vi "Rear Rocket to Score.vi"() -> (4 "path":cluster{"X":dbl, "Y":dbl}[](array[cluster])=[{"X"=300.0, "Y"=62.0}, {"X"=299.67796585022535, "Y"=61.06513991194655}, {"X"=299.35531113454925, "Y"=60.131107487190775}, {"X"=299.0313812985895, "Y"=59.19877965387899}, {"X"=298.7054549995574, "Y"=58.26912580374255}, {"X"=298.376704877581, "Y"=57.343252442862465}, {"X"=298.04415663192685, "Y"=56.42246009840396}, {"X"=297.70664011718065, "Y"=55.50831518041174}, {"X"=297.3627267868247, "Y"=54.602736376469785}, {"X"=297.010650930695, "Y"=53.708096849775444}, {"X"=296.64821357013733, "Y"=52.82734746493497}, {"X"=296.2726661277642, "Y"=51.96416944345233}, {"X"=295.88056891520927, "Y"=51.123167538744006}, {"X"=295.4676069213577, "Y"=50.31010763033021}, {"X"=295.0283908833696, "Y"=49.532242809593704}, {"X"=294.5560954613462, "Y"=48.7986359651749}, {"X"=294.0284648626625, "Y"=48.0784796591909}, {"X"=293.4567720099731, "Y"=47.36905297576079}, {"X"=292.85006167096424, "Y"=46.66825385588848}, {"X"=292.21553026302087, "Y"=45.9744402337975}, {"X"=291.5588656657838, "Y"=45.28630800332636}, {"X"=290.8846000891376, "Y"=44.60285095835355}, {"X"=290.196364261339, "Y"=43.92332453368775}, {"X"=289.49705315511903, "Y"=43.24719469139753}, {"X"=288.7889647280253, "Y"=42.574098303654296}, {"X"=288.0739306067003, "Y"=41.90382692056283}, {"X"=287.35342424819305, "Y"=41.23632388947038}, {"X"=286.6286381471462, "Y"=40.57168374443791}, {"X"=285.90053857777383, "Y"=39.91015312672445}, {"X"=285.1699127607743, "Y"=39.2521400561977}, {"X"=284.43740364738807, "Y"=38.59822952777461}, {"X"=283.70358294426364, "Y"=37.949238228876666}, {"X"=282.9688855497176, "Y"=37.30619626764946}, {"X"=282.2338323047616, "Y"=36.670539509494894}, {"X"=281.4987765734628, "Y"=36.04397819113178}, {"X"=280.7641553421933, "Y"=35.42878692701308}, {"X"=280.03044421363336, "Y"=34.827824744652226}, {"X"=279.2981146207875, "Y"=34.24466579102106}, {"X"=278.56770897603565, "Y"=33.68383375390436}, {"X"=277.8399028708086, "Y"=33.151044376258625}, {"X"=277.0852340691614, "Y"=32.62621063659758}, {"X"=276.3096142473145, "Y"=32.10793481435018}, {"X"=275.51783999700325, "Y"=31.59516350001117}, {"X"=274.71386264087107, "Y"=31.087138412194943}, {"X"=273.9010019494029, "Y"=30.583354256294154}, {"X"=273.0821128441466, "Y"=30.08352650030417}, {"X"=272.2597284445897, "Y"=29.58757798169254}, {"X"=271.43618730520296, "Y"=29.095626058533444}, {"X"=270.6137768577266, "Y"=28.60801853264354}, {"X"=269.7948293153701, "Y"=28.125304207113395}, {"X"=268.9818874214875, "Y"=27.648321209906022}, {"X"=268.17779535712015, "Y"=27.17819420680734}, {"X"=267.3858611746366, "Y"=26.716401759600387}, {"X"=266.61003761727807, "Y"=26.26486982962313}, {"X"=265.85512070414063, "Y"=25.82606549423999}, {"X"=265.1270026053729, "Y"=25.40312036911472}, {"X"=264.4329896907217, "Y"=25.0}], 6 "Reverse Path?":bool)   [LabVIEW 2018]
uses:
  AutonBuilder/Typedef/Data Point.ctl
panel:
  in  "Data Points":T1[](array[typedef])=[{"X"=300.0, "Y"=62.0, "Theta"=0.0, "Speed %"=0.0, "Disabled?"=FALSE}, {"X"=295.60824742268045, "Y"=48.54355400696864, "Theta"=0.0, "Speed %"=0.0, "Disabled?"=FALSE}, {"X"=278.35051546391753, "Y"=33.0, "Theta"=0.0, "Speed %"=0.0, "Disabled?"=FALSE}, {"X"=264.4329896907217, "Y"=25.0, "Theta"=0.0, "Speed %"=0.0, "Disabled?"=FALSE}]
  out "Graph":cluster{dbl[], dbl[]}[](graph)=[{[280.5, 314.0, 314.0, 280.5, 280.5], [76.25, 76.25, 47.75, 47.75, 76.25]}, {[300.0, 295.60824742268045, 278.35051546391753, 264.4329896907217], [62.0, 48.54355400696864, 33.0, 25.0]}, {[300.0, 299.67796585022535, 299.35531113454925, 299.0313812985895, 298.7054549995574, 298.376704877581, 298.04415663192685, 297.70664011718065, 297.3627267868247, 297.010650930695, 296.64821357013733, 296.2726661277642, 295.88056891520927, 295.4676069213577, 295.0283908833696, 294.5560954613462, 294.0284648626625, 293.4567720099731, 292.85006167096424, 292.21553026302087, 291.5588656657838, 290.8846000891376, 290.196364261339, 289.49705315511903, 288.7889647280253, 288.0739306067003, 287.35342424819305, 286.6286381471462, 285.90053857777383, 285.1699127607743, 284.43740364738807, 283.70358294426364, 282.9688855497176, 282.2338323047616, 281.4987765734628, 280.7641553421933, 280.03044421363336, 279.2981146207875, 278.56770897603565, 277.8399028708086, 277.0852340691614, 276.3096142473145, 275.51783999700325, 274.71386264087107, 273.9010019494029, 273.0821128441466, 272.2597284445897, 271.43618730520296, 270.6137768577266, 269.7948293153701, 268.9818874214875, 268.17779535712015, 267.3858611746366, 266.61003761727807, 265.85512070414063, 265.1270026053729, 264.4329896907217], [62.0, 61.06513991194655, 60.131107487190775, 59.19877965387899, 58.26912580374255, 57.343252442862465, 56.42246009840396, 55.50831518041174, 54.602736376469785, 53.708096849775444, 52.82734746493497, 51.96416944345233, 51.123167538744006, 50.31010763033021, 49.532242809593704, 48.7986359651749, 48.0784796591909, 47.36905297576079, 46.66825385588848, 45.9744402337975, 45.28630800332636, 44.60285095835355, 43.92332453368775, 43.24719469139753, 42.574098303654296, 41.90382692056283, 41.23632388947038, 40.57168374443791, 39.91015312672445, 39.2521400561977, 38.59822952777461, 37.949238228876666, 37.30619626764946, 36.670539509494894, 36.04397819113178, 35.42878692701308, 34.827824744652226, 34.24466579102106, 33.68383375390436, 33.151044376258625, 32.62621063659758, 32.10793481435018, 31.59516350001117, 31.087138412194943, 30.583354256294154, 30.08352650030417, 29.58757798169254, 29.095626058533444, 28.60801853264354, 28.125304207113395, 27.648321209906022, 27.17819420680734, 26.716401759600387, 26.26486982962313, 25.82606549423999, 25.40312036911472, 25.0]}, {[302.86466642002404, 286.2049296430795, 285.8863016143085, 285.5706984813838, 285.25794442422927, 284.9480898615065, 284.64144909579124, 284.33869923581494, 284.04105177421627, 283.75052314685786, 283.470370216165, 283.20581673896623, 282.9652805494417, 282.76247671309693, 282.6198192416317, 282.57443861469056, 282.5335104549795, 282.3611354437252, 282.0765565739421, 281.70003519026403, 281.2496358321106, 280.7403468790285, 280.18445756578194, 279.59201059374533, 278.9711237054457, 278.3283352571779, 277.6689893589384, 276.99757110000064, 276.31795020342184, 275.6335640622988, 274.94761135851314, 274.2631927751518, 273.5836926739073, 272.9127122773153, 272.254686832191, 271.6151631816832, 271.0009291706447, 270.42133708095275, 269.8892351862872, 269.4225804954357, 268.9491661733871, 268.39249314054535, 267.771752324279, 267.101785832785, 266.39415115658835, 265.65798842977506, 264.9007111618025, 264.12836881993337, 263.34630014905264, 262.55887615613375, 261.7705371414297, 260.98538541760917, 260.2076610195241, 259.44210017421875, 258.6940092313346, 257.96945960930367, 257.27563161638744], [48.040910262413725, 65.7062384199441, 64.78387897778246, 63.87558605297041, 62.983673430656296, 62.11135465968407, 61.262907464176386, 60.44396676782252, 59.66193343316213, 58.92647889369578, 58.25016449468687, 57.64923294797633, 57.14461474262013, 56.76318181176808, 56.53865771394094, 56.51241579149808, 56.50038699454487, 56.31049297107146, 55.99531598307725, 55.59144929976111, 55.124106549571465, 54.61067923471754, 54.06355255476597, 53.49183386793153, 52.90233618120884, 52.30026242910942, 51.689754947060386, 51.07430472842981, 50.45702470306093, 49.84083938619493, 49.228673653680666, 48.62357818294111, 48.02909954446028, 47.449186058757896, 46.88876057047503, 46.353915871191504, 45.85190557202472, 45.39210139335965, 44.986337577422795, 44.64935660149614, 44.32522338107097, 43.95621289096325, 43.55595886513926, 43.13366432914706, 42.69573185833495, 42.2467857954081, 41.79033851493417, 41.32911652472306, 40.86551755523709, 40.401438854360336, 39.93892441472516, 39.479890807765415, 39.026395363706875, 38.58084209381681, 38.14600796464324, 37.72513636729536, 37.32212341261694]}, {[297.13533357997596, 313.1510020573712, 312.82432065479003, 312.49206411579524, 312.1529655748855, 311.8053198936555, 311.44686416806246, 311.07458099854637, 310.6844017994331, 310.2707787145322, 309.82605692410965, 309.33951551656213, 308.79585728097686, 308.17273712961844, 307.43696252510745, 306.53775230800187, 305.52341927034547, 304.55240857622107, 303.62356676798635, 302.7310253357777, 301.868095499457, 301.02885329924675, 300.20827095689606, 299.40209571649274, 298.6068057506049, 297.81952595622266, 297.0378591374477, 296.25970519429177, 295.4831269521258, 294.70626145924984, 293.927195936263, 293.14397311337547, 292.35407842552786, 291.55495233220796, 290.7428663147346, 289.9131475027034, 289.059959256622, 288.1748921606222, 287.2461827657841, 286.2572252461815, 285.2213019649357, 284.2267353540837, 283.2639276697275, 282.3259394489571, 281.4078527422174, 280.5062372585181, 279.6187457273769, 278.74400579047256, 277.8812535664005, 277.0307824746065, 276.1932377015453, 275.3702052966311, 274.5640613297491, 273.7779750603374, 273.0162321769467, 272.2845456014422, 271.5903477650559], [75.95908973758628, 56.424041403949005, 55.47833599659909, 54.52197325478756, 53.5545781768288, 52.57515022604086, 51.58201273263153, 50.57266359300096, 49.54353931977744, 48.48971480585511, 47.40453043518306, 46.279105938928325, 45.101720334867885, 43.85703344889234, 42.525827905246466, 41.08485613885173, 39.656572323836926, 38.427612980450114, 37.34119172869971, 36.357431167833894, 35.44850945708126, 34.59502268198956, 33.783096512609525, 33.00255551486353, 32.24586042609975, 31.50739141201624, 30.782892831880368, 30.069062760446013, 29.363281550387974, 28.663440726200477, 27.96778540186856, 27.274898274812223, 26.583292990838643, 25.891892960231893, 25.199195811788528, 24.503657982834653, 23.803743917279732, 23.097230188682474, 22.381329930385924, 21.652732151021116, 20.927197892124184, 20.25965673773711, 19.63436813488308, 19.040612495242826, 18.470976654253352, 17.92026720520024, 17.38481744845091, 16.862135592343826, 16.35051951004999, 15.849169559866455, 15.357718005086886, 14.876497605849265, 14.406408155493898, 13.948897565429451, 13.506123023836741, 13.081104370934082, 12.677876587383059]}, {[], []}, {[], []}, {[], []}, {[], []}, {[], []}, {[], []}, {[], []}, {[], []}, {[], []}, {[], []}, {[], []}, {[], []}, {[], []}, {[], []}, {[], []}, {[], []}, {[], []}, {[], []}, {[], []}, {[], []}]
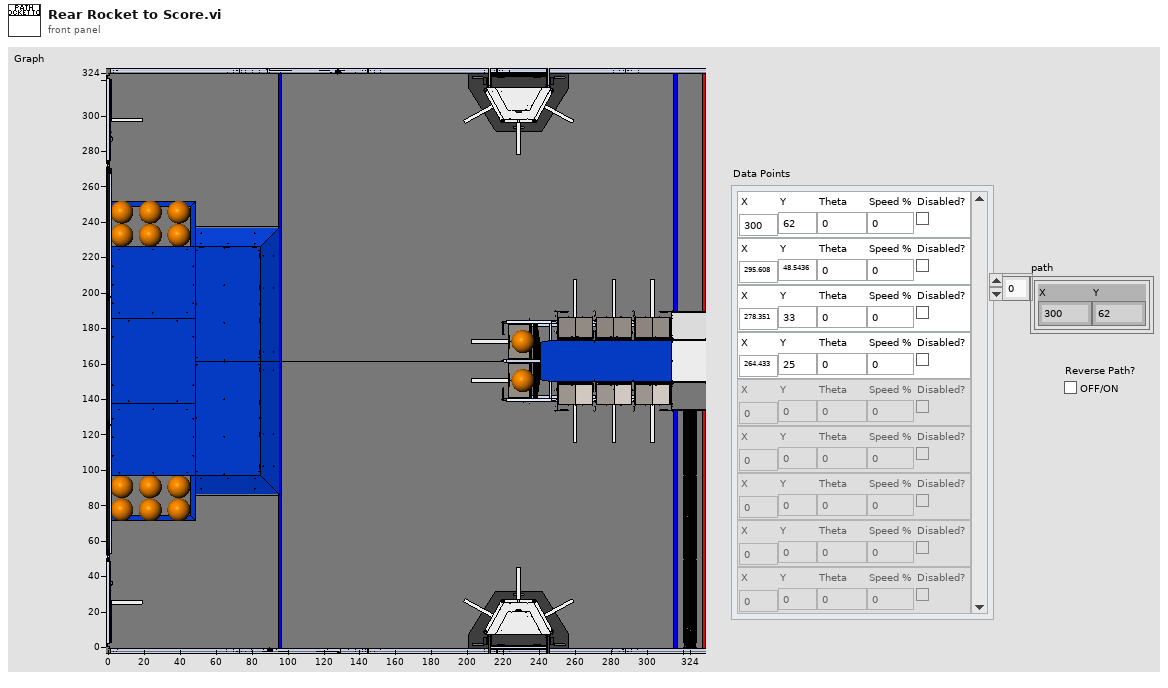
[diagram p1: front panel]
types:
  T1 = typedef "Data Point.ctl" = cluster{"X":dbl, "Y":dbl, "Theta":dbl, "Speed %":dbl, "Disabled?":bool}
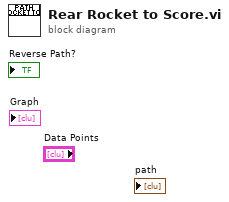
[diagram p0: block diagram]
diagram:
